vi "configServer.vi"(8 "error in (no error)":errorcluster, 10 "ServerConfiguration":T1={"cmdServerPort"=8888, "telServerPort"=8889, "serverTimeout (ms)"=100, "serverBytesToRead"=32768, "maxSizeQueueTcpClientFromDds"=1000, "EnqueueOptions"=enum."lossy enqueue", "queueTcpClientFromDdsTimeout (ms)"=50, "maxSizeQueueTcpClient"=1000, "timeoutInMs"=100}, 11 "tcpServer in":refnum<class "TcpServer.lvclass">) -> (0 "error out":errorcluster, 3 "tcpServer out":refnum<class "TcpServer.lvclass">)   [LabVIEW 2018, in "TcpServer.lvclass"]
doc: "Configure the TCP Server Command and TCP Server Telemetry."
uses:
  TcpServer.lvclass
  configServerTypeDef.ctl
  TcpServerTel/typedef/enqueueOptionsTypeDef.ctl
  TcpServer.lvclass/TcpServer.ctl
  TcpServerBase/TcpServerBase.lvclass/TcpServerBase.ctl
  TcpServerTel/TcpServerTel.lvclass/TcpServerTel.ctl
  TcpServerCmd/TcpServerCmd.lvclass
  home/pcortes/github/ts_labview_tcp_json/src/TcpServerBase/TcpServerBase.lvclass
  TcpServerTel/TcpServerTel.lvclass
  TcpServerBase/TcpServerBase.lvclass
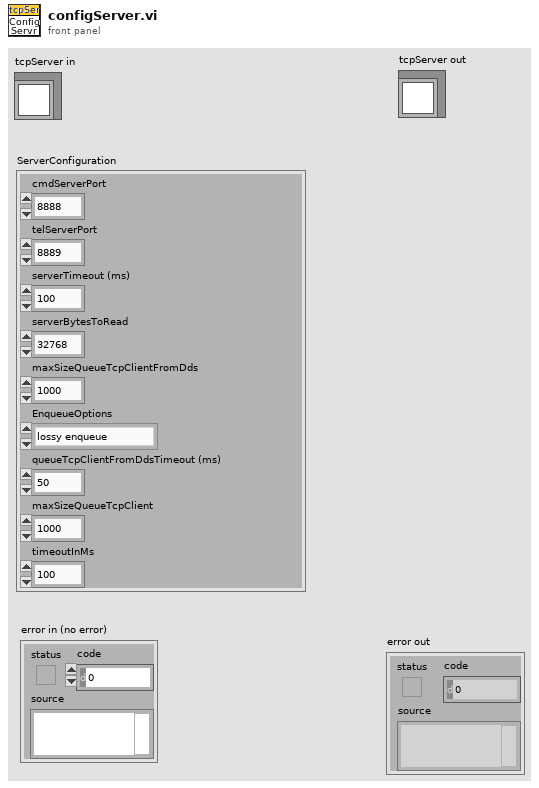
[diagram p1: front panel]
types:
  T1 = typedef "TcpServer.lvclass/configServerTypeDef.ctl" = cluster{"cmdServerPort":u16, "telServerPort":u16, "serverTimeout (ms)":i32, "serverBytesToRead":i32, "maxSizeQueueTcpClientFromDds":i32, "EnqueueOptions":T2, "queueTcpClientFromDdsTimeout (ms)":i32, "maxSizeQueueTcpClient":i32, "timeoutInMs":i32}
  T2 = typedef "TcpServerTel.lvclass/enqueueOptionsTypeDef.ctl" = enum16{"lossy enqueue", "normal enqueue"}
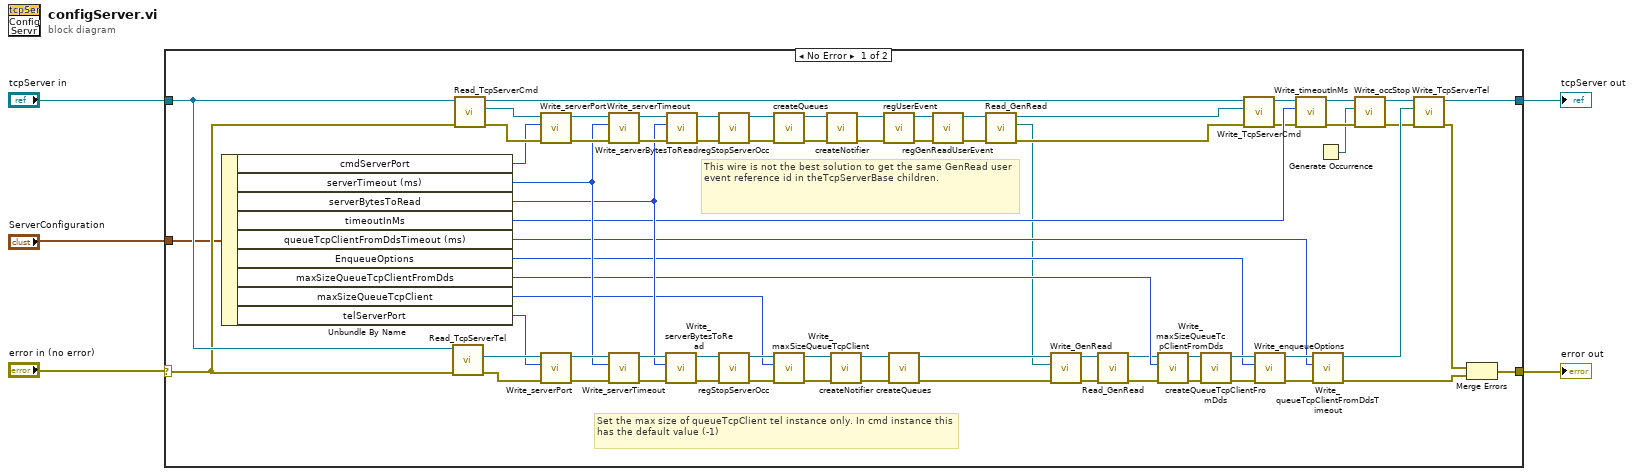
[diagram p0: block diagram]
diagram:
  n1 = case shown="No Error" "error in (no error)" {
    selector: "error in (no error)" -> [w68 w78]
    tunnel: "tcpServer in" -> [w70 w79]
    tunnel: "ServerConfiguration" -> [w59 _]
    tunnel: [w56 w79] -> w3
    tunnel: [w63 w78] -> w2
    frame No Error {
      # "This wire is not the best solution to get the same GenRead user event reference id in theTcpServerBase children."
      # "Set the max size of queueTcpClient tel instance only. In cmd instance this has the default value (-1)"
      n2 = Unbundle By Name(w59) -> ("cmdServerPort"=w66:u16, "serverTimeout (ms)"=w58:i32, "serverBytesToRead"=w57:i32, "timeoutInMs"=w35:i32, "queueTcpClientFromDdsTimeout (ms)"=w41:i32, "EnqueueOptions"=w45:T2, "maxSizeQueueTcpClientFromDds"=w38:i32, "maxSizeQueueTcpClient"=w37:i32, "telServerPort"=w48:u16)
      n3 = call "Read_TcpServerTel.vi"("error in (no error)"=w68, "TcpServer in"=w70) -> ("error out"=w67:errorcluster, "TcpServerTel.lvclass"=w69:refnum<class "TcpServerTel.lvclass">)  [unwired: 7 in, 1 out]
      n4 = call "Read_TcpServerCmd.vi"("error in (no error)"=w68, "TcpServer in"=w70) -> ("error out"=w71:errorcluster, "TcpServerCmd.lvclass"=w72:refnum<class "TcpServerCmd.lvclass">, "TcpServer out"=w65:refnum<class "TcpServer.lvclass">)  [unwired: 7 in]
      n5 = call "Write_serverPort.vi"("error in (no error)"=w71, "serverPort"=w66, "TcpServerBase in"=w72) -> ("error out"=w76:errorcluster, "TcpServerBase out"=w77:refnum<class "TcpServerCmd.lvclass">)  [unwired: 7 in]
      n6 = call "Write_serverPort.vi"("error in (no error)"=w67, "serverPort"=w48, "TcpServerBase in"=w69) -> ("error out"=w64:errorcluster, "TcpServerBase out"=w61:refnum<class "TcpServerTel.lvclass">)  [unwired: 7 in]
      n7 = call "Write_serverTimeout.vi"("error in (no error)"=w76, "serverTimeout"=w58, "TcpServerBase in"=w77) -> ("error out"=w74:errorcluster, "TcpServerBase out"=w75:refnum<class "TcpServerCmd.lvclass">)  [unwired: 7 in]
      n8 = call "Write_serverTimeout.vi"("error in (no error)"=w64, "serverTimeout"=w58, "TcpServerBase in"=w61) -> ("error out"=w62:errorcluster, "TcpServerBase out"=w60:refnum<class "TcpServerTel.lvclass">)  [unwired: 7 in]
      n9 = call "Write_serverBytesToRead.vi"("error in (no error)"=w62, "serverBytesToRead"=w57, "TcpServerBase in"=w60) -> ("error out"=w20:errorcluster, "TcpServerBase out"=w21:refnum<class "TcpServerTel.lvclass">)  [unwired: 7 in]
      n10 = call "Write_serverBytesToRead.vi"("error in (no error)"=w74, "serverBytesToRead"=w57, "TcpServerBase in"=w75) -> ("error out"=w22:errorcluster, "TcpServerBase out"=w23:refnum<class "TcpServerCmd.lvclass">)  [unwired: 7 in]
      n11 = call "regStopServerOcc.vi"("error in (no error)"=w22, "tcpServerBase in"=w23) -> ("error out"=w54:errorcluster, "tcpServerBase out"=w53:refnum<class "TcpServerCmd.lvclass">)  [unwired: 8 in]
      n12 = call "regStopServerOcc.vi"("error in (no error)"=w20, "tcpServerBase in"=w21) -> ("error out"=w52:errorcluster, "tcpServerBase out"=w49:refnum<class "TcpServerTel.lvclass">)  [unwired: 8 in]
      n13 = call "createQueues.vi"("error in (no error)"=w54, "tcpServerBase in"=w53) -> ("error out"=w73:errorcluster, "tcpServerBase out"=w29:refnum<class "TcpServerCmd.lvclass">)  [unwired: 8 in]
      n14 = call "Write_maxSizeQueueTcpClient.vi"("error in (no error)"=w52, "maxSizeQueueTcpClient"=w37, "TcpServerBase in"=w49) -> ("error out"=w50:errorcluster, "TcpServerBase out"=w27:refnum<class "TcpServerTel.lvclass">)  [unwired: 7 in]
      n15 = call "createNotifier.vi"("error in (no error)"=w73, "tcpServerBase in"=w29) -> ("error out"=w30:errorcluster, "tcpServerBase out"=w19:refnum<class "TcpServerCmd.lvclass">)  [unwired: 8 in]
      n16 = call "createNotifier.vi"("error in (no error)"=w50, "tcpServerBase in"=w27) -> ("error out"=w28:errorcluster, "tcpServerBase out"=w26:refnum<class "TcpServerTel.lvclass">)  [unwired: 8 in]
      n17 = call "regUserEvent.vi"("error in (no error)"=w30, "tcpServerCmd in"=w19) -> ("error out"=w18:errorcluster, "tcpServerCmd out"=w16:refnum<class "TcpServerCmd.lvclass">)  [unwired: 8 in]
      n18 = call "createQueues.vi"("error in (no error)"=w28, "tcpServerBase in"=w26) -> ("error out"=w11:errorcluster, "tcpServerBase out"=w10:refnum<class "TcpServerTel.lvclass">)  [unwired: 8 in]
      n19 = call "regGenReadUserEvent.vi"("error in (no error)"=w18, "TcpServerBase in"=w16) -> ("error out"=w17:errorcluster, "TcpServerBase out"=w13:refnum<class "TcpServerCmd.lvclass">)  [unwired: 8 in]
      n20 = call "Read_GenRead.vi"("error in (no error)"=w17, "TcpServerBase in"=w13) -> ("error out"=w14:errorcluster, "GenRead"=w9:refnum<user-event>, "TcpServerBase out"=w12:refnum<class "TcpServerCmd.lvclass">)  [unwired: 7 in]
      n21 = call "Write_GenRead.vi"("error in (no error)"=w11, "GenRead"=w9, "TcpServerBase in"=w10) -> ("error out"=w15:errorcluster, "TcpServerBase out"=w7:refnum<class "TcpServerTel.lvclass">)  [unwired: 7 in]
      n22 = call "Read_GenRead.vi"("error in (no error)"=w15, "TcpServerBase in"=w7) -> ("error out"=w8:errorcluster, "TcpServerBase out"=w6:refnum<class "TcpServerTel.lvclass">)  [unwired: 7 in, 1 out]
      n23 = call "Write_maxSizeQueueTcpClientFromDds.vi"("error in (no error)"=w8, "maxSizeQueueTcpClientFromDds"=w38, "TcpServerTel in"=w6) -> ("error out"=w40:errorcluster, "TcpServerTel out"=w39:refnum<class "TcpServerTel.lvclass">)  [unwired: 7 in]
      n24 = call "createQueueTcpClientFromDds.vi"("error in (no error)"=w40, "tcpServerTel in"=w39) -> ("error out"=w51:errorcluster, "tcpServerTel out"=w46:refnum<class "TcpServerTel.lvclass">)  [unwired: 8 in]
      n25 = call "Write_TcpServerCmd.vi"("error in (no error)"=w14, "TcpServerCmd.lvclass"=w12, "TcpServer in"=w65) -> ("error out"=w24:errorcluster, "TcpServer out"=w25:refnum<class "TcpServer.lvclass">)  [unwired: 7 in]
      n26 = call "Write_enqueueOptions.vi"("error in (no error)"=w51, "EnqueueOptions"=w45, "TcpServerTel in"=w46) -> ("error out"=w47:errorcluster, "TcpServerTel out"=w43:refnum<class "TcpServerTel.lvclass">)  [unwired: 7 in]
      n27 = call "Write_timeoutInMs.vi"("error in (no error)"=w24, "timeoutInMs"=w35, "TcpServer in"=w25) -> ("error out"=w36:errorcluster, "TcpServer out"=w33:refnum<class "TcpServer.lvclass">)  [unwired: 7 in]
      n28 = call "Write_queueTcpClientFromDdsTimeout.vi"("error in (no error)"=w47, "queueTcpClientFromDdsTimeout"=w41, "TcpServerTel in"=w43) -> ("error out"=w44:errorcluster, "TcpServerTel out"=w42:refnum<class "TcpServerTel.lvclass">)  [unwired: 7 in]
      n29 = Generate Occurrence() -> (w31:refnum<k4>)
      n30 = call "Write_occStop.vi"("error in (no error)"=w36, "occStop"=w31, "TcpServer in"=w33) -> ("error out"=w34:errorcluster, "TcpServer out"=w32:refnum<class "TcpServer.lvclass">)  [unwired: 7 in]
      n31 = call "Write_TcpServerTel.vi"("error in (no error)"=w34, "TcpServerTel.lvclass"=w42, "TcpServer in"=w32) -> ("error out"=w55:errorcluster, "TcpServer out"=w56:refnum<class "TcpServer.lvclass">)  [unwired: 7 in]
      n32 = Merge Errors(w55, w44) -> (w63:errorcluster)
    }
    frame Error {
    }
  }
  "error out" <- w2
  "tcpServer out" <- w3
